vi "NIP Data.vi"(10 "index (row)":i32=2, 11 "file path (dialog if empty)":path=path "C:/Users/ATMA/Desktop/data.txt") -> (2 "Data":string[][](array[string]), 3 "file path (dialog if empty) 2":path)   [LabVIEW 2015]
uses:
  Galobal variable_TI.vi
  <vilib>/Utility/file.llb/Read Delimited Spreadsheet (string).vi
panel:
  out "first row":string[][](array[string])
  out "error out":errorcluster
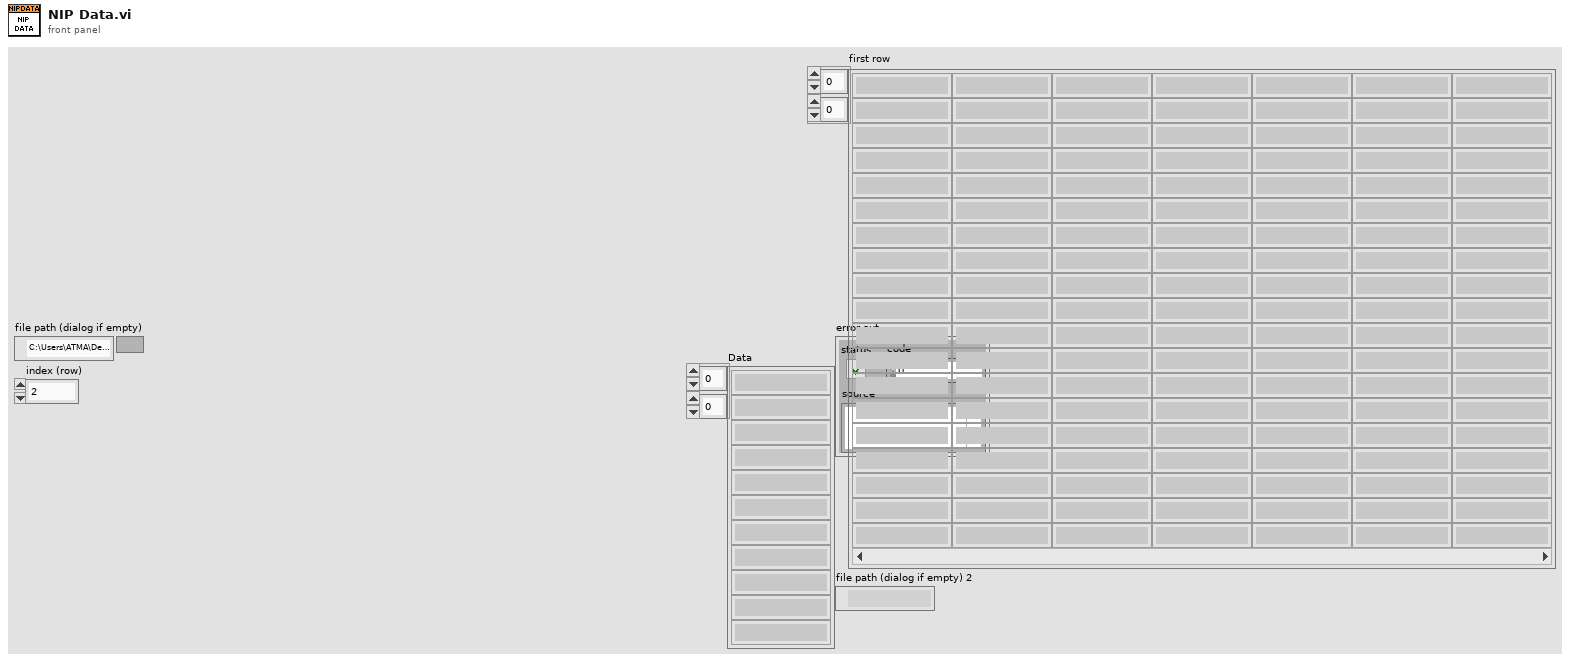
[diagram p1: front panel]
types:
  T1 = cluster{"To-A":timestamp, "From-A":timestamp, "From-B":timestamp, "To-B":timestamp, "From-C 1":timestamp, "To-C 1":timestamp, "From-C 2":timestamp, "To-C 2":timestamp, "Shift":string}
  T2 = cluster{"Stn Name":string, "date":string, "time":string, "Operator id":string, "Shift":string, "Error Code":string, "Fail count":string, "Rework":string, "NA":string, "Tested":string}
  T3 = cluster{"To-A":timestamp, "From-A":timestamp, "From-B":timestamp, "To-B":timestamp, "From-C 1":timestamp, "To-C 1":timestamp, "From-C 2":timestamp, "To-C 2":timestamp}
  T4 = cluster{"No. Fail Coun t":string, "Rework Status Count 0\\1":string, "NA Count Max =3 ":string, "Testesd Count  0/1":string, "Error code":string}
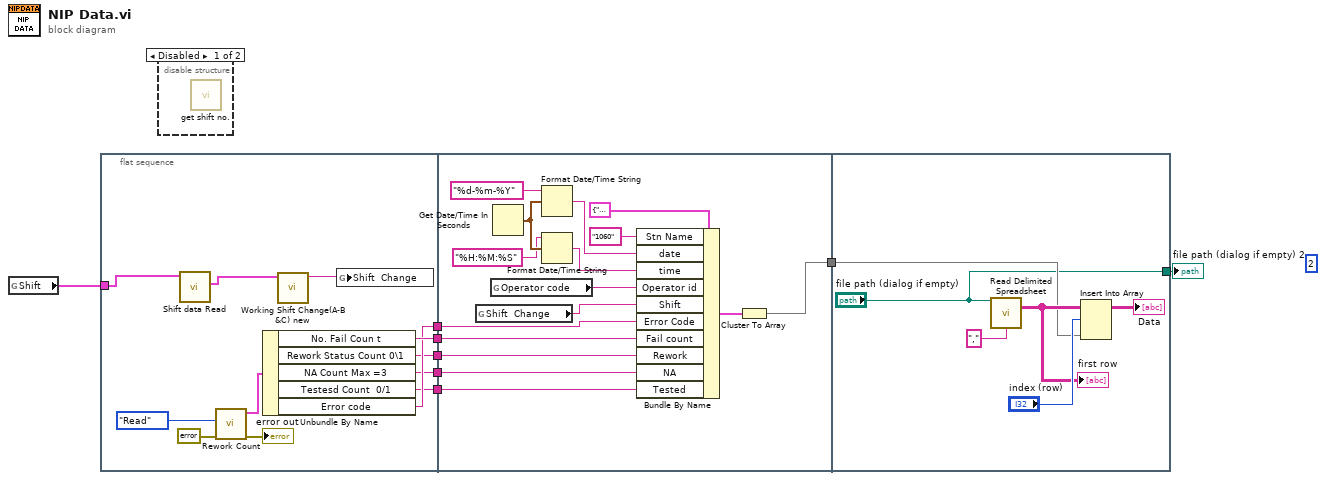
[diagram p0: block diagram]
diagram:
  (unwired) 2 ("disabled index (col)")
  n1 = global read "Galobal variable_TI.vi" "Shift"() -> (w1:T1)
  n2 = flat-sequence {
    tunnel: [w16] -> w8
    tunnel: [w15] -> w7
    tunnel: [w14] -> w6
    tunnel: [w13] -> w5
    tunnel: [w12] -> w4
    tunnel: w1 -> [w9]
    tunnel: w8 -> [w26]
    tunnel: w7 -> [w25]
    tunnel: w6 -> [w24]
    tunnel: w5 -> [w23]
    tunnel: w4 -> [w22]
    tunnel: [w21] -> w3
    tunnel: w3 -> [w39]
    tunnel: ["file path (dialog if empty)"] -> w2
    frame #0 {
      n3 = call "Shift data Read.vi"("input cluster"=w9) -> ("output cluster"=w11:T3)  [unwired: 10 in]
      n4 = call "Rework Count.vi"("error in"=errorcluster {"status"=FALSE, "code"=0, "source"=""}, "Read /Write"=enum16{"Write", "Read"}."Read") -> ("error out"=→"error out":errorcluster, "data"=w18:T4)  [unwired: 8 in]
      n5 = Unbundle By Name(w18) -> ("No. Fail Coun t"=w16:string, "Rework Status Count 0\\1"=w14:string, "NA Count Max =3"=w13:string, "Testesd Count  0/1"=w12:string, "Error code"=w15:string)
      n6 = call "Working Shift Change(A-B &C) new.vi"("input cluster"=w11) -> ("Shift Change"=w10:string)  [unwired: 10 in]
      n7 = global write "Galobal variable_TI.vi" "Shift  Change"(w10) -> ()
    }
    frame #1 {
      n8 = global read "Galobal variable_TI.vi" "Shift  Change"() -> (w27:string)
      n9 = global read "Galobal variable_TI.vi" "Operator code"() -> (w28:string)
      n10 = Get Date/Time In Seconds() -> (seconds since 1Jan1904=w34:timestamp)
      n11 = Format Date/Time String(time format string (%c)="%d-%m-%Y", seconds (now)=w34) -> (date/time string=w35:string)  [unwired: 1 in]
      n12 = Format Date/Time String(time format string (%c)="%H:%M:%S", seconds (now)=w34) -> (date/time string=w32:string)  [unwired: 1 in]
      n13 = Bundle By Name(cluster=T2 {"Stn Name"="", "date"="", "time"="", "Operator id"="", "Shift"="", "Error Code"="", "Fail count"="", "Rework"="", "NA"="", "Tested"=""} ("Write Data"), "Stn Name"="1060", "date"=w35, "time"=w32, "Operator id"=w28, "Shift"=w27, "Error Code"=w25, "Fail count"=w26, "Rework"=w24, "NA"=w23, "Tested"=w22) -> (w31:T2)
      n14 = Cluster To Array(cluster=w31) -> (array=w21:string[])
    }
    frame #2 {
      n15 = call-poly <vilib>:"Read Delimited Spreadsheet.vi"("file path (dialog if empty)"="file path (dialog if empty)", "delimiter (\\t)"="," ("delimiter (\\t)")) -> ("all rows"=w40:string[][])  [unwired: 8 in, 5 out]
      "first row" <- w40
      n16 = Insert Into Array(array=w40, index (row)="index (row)", new element=w39) -> (→"Data":string[][])  [unwired: 1 in]
    }
  }
  n17 = disable-structure shown="Disabled" {
    frame Disabled {
      n18 = call "get shift no..vi"() -> ()  [unwired: 11 in, 1 out]
    }
    frame Enabled {
    }
  }
  "file path (dialog if empty) 2" <- w2
